vi "Teleop.vi"(10 "Match Info":T2={"Autonomous Elapsed Seconds"=0.0, "TeleOp Elapsed Seconds"=0.0, "Disabled Elapsed Seconds"=0.0, "Visited Autonomous"=FALSE, "Visited TeleOp"=FALSE, "Visited Disabled"=FALSE, "Autonomous Settings"={"Autonomous Style"=enum."Independent", "VI Refnum"=refnum}}, 11 "Call Context":T1) -> ()   [LabVIEW 2013]
doc: "This VI is called for each TeleOp packet received from the DS where the robot is not disabled. It is often used to read from the joysticks and update I/O or to update setpoints for timed control loops. It should complete and return within 20 milliseconds or it may miss DS packets."
uses:
  <vilib>/Rock Robotics/WPI/DriverStation/WPI_DriverStationMatch Info.ctl
  <vilib>/Rock Robotics/WPI/DriverStation/WPI_DriverStationDerivedRobotMode.ctl
  Robot Global Data.vi
  <vilib>/Rock Robotics/WPI/Solenoid/Deprecated/WPI_SolenoidSetBool.vi
  <vilib>/Rock Robotics/WPI/Joystick/WPI_JoystickGetSetRefNum.vi
  <vilib>/Rock Robotics/WPI/Compressor/WPI_CompressorGetSetRefNum.vi
  <vilib>/Rock Robotics/WPI/RobotDrive/WPI_RobotDriveGetSetRefNum.vi
panel:
  in  "Uncock tension":dbl=0.15
  in  "Manual Tension Power":dbl=0.7
  out "hot?":bool
  out "shouldTurnRight":bool
  in  "Ball In Delay":dbl=1.75
  out "Arm Half Out":bool
  out "Timings":cluster{"Call Name":string, "Delta (ms)":u32}[](array[cluster])
  out "Right":dbl
  out "Left":dbl
  out "Encoders":dbl
  out "Angular Rate":dbl
  out "Angle":dbl
  out "Numeric 1":dbl(slide) scale=0.0..100.0
  out "Boolean 2":bool
  out "Boolean 1":bool
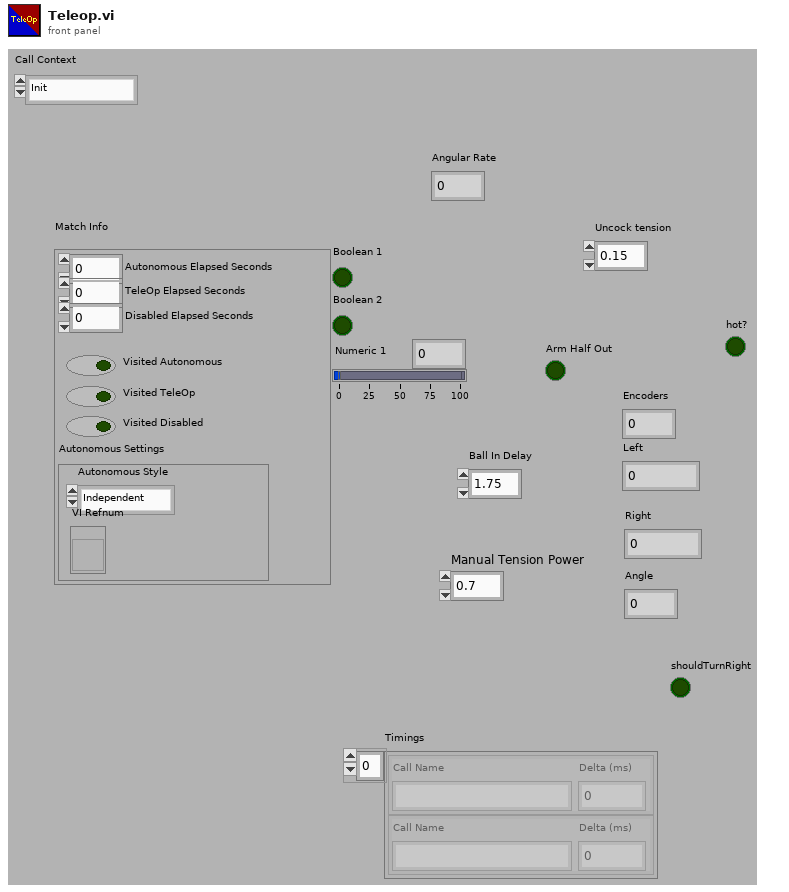
[diagram p1: front panel]
types:
  T1 = typedef "WPI_DriverStationDerivedRobotMode.ctl" = enum16{"Init", "Execute", "Stop"}
  T2 = typedef "WPI_DriverStationMatch Info.ctl" = cluster{"Autonomous Elapsed Seconds":dbl, "TeleOp Elapsed Seconds":dbl, "Disabled Elapsed Seconds":dbl, "Visited Autonomous":bool, "Visited TeleOp":bool, "Visited Disabled":bool, "Autonomous Settings":cluster{"Autonomous Style":enum16{"Iterative", "Independent"}, "VI Refnum":refnum<vi>}}
  T3 = typedef "WPI_JoystickDevRef.ctl" = cluster{"Device":T4}
  T4 = typedef "WPI_JoystickDeviceEnum.ctl" = enum16{"USB 1", "USB 2", "USB 3", "USB 4", "Kinect 1", "Kinect 2"}
  T5 = typedef "WPI_RobotDriveDevRef.ctl" = cluster{"DevStatus":errorcluster, "Motors[]":T6[], "Square Inputs":bool, "Max Output":dbl, "Isochronous":bool}
  T6 = typedef "WPI_MotorControlDeviceRef.ctl" = cluster{"DeviceStatus":errorcluster, "Type":enum16{"PWM", "CAN"}, "PWM":cluster{"Digital Module":T7, "PWM Channel":T8, "DeadBand":T9}, "CAN":cluster{"Device Number":u8, "Control Mode":T10, "Semaphore":T11, "Max Vout":dbl}, "Invert":bool, "TransformRef":T12, "InvTransformRef":T12}
  T7 = typedef "FPGA_TypedefDigitalModule.ctl" = enum16{"Digital Module 1", "Digital Module 2"}
  T8 = typedef "FPGA_DIOPWMChannel.ctl" = enum8{"PWM 1", "PWM 2", "PWM 3", "PWM 4", "PWM 5", "PWM 6", "PWM 7", "PWM 8", "PWM 9", "PWM 10", "Invalid"}
  T9 = typedef "WPI_PWMDeadband.ctl" = cluster{"Name":string, "maxPositivePwm":i32, "minPositivePwm":i32, "centerPwm":i32, "maxNegativePwm":i32, "minNegativePwm":i32, "angularRange":u16}
  T10 = typedef "WPI_CANJaguar_ControlMode.ctl" = enum8{"Percent VBus", "Current", "Speed", "Position", "Voltage"}
  T11 = typedef "Semaphore RefNum" = refnum<k1>
  T12 = typedef "WPI_PWMTransform_ConPane.ctl" = refnum<vi>
  T13 = typedef "WPI_JoystickButtonState.ctl" = cluster{"Button 1":bool, "Button 2":bool, "Button 3":bool, "Button 4":bool, "Button 5":bool, "Button 6":bool, "Button 7":bool, "Button 8":bool, "Button 9":bool, "Button 10":bool, "Button 11":bool, "Button 12":bool}
  T14 = cluster{"axis 1 (x)":dbl, "axis 2 (y)":dbl, "axis 3 (throttle)":dbl, "axis 4":dbl, "axis 5":dbl, "axis 6":dbl}
  T15 = typedef "WPI_CompressorDevRef.ctl" = cluster{"DevStatus":errorcluster, "DigitalInputDevRef":T16, "RelayDevRef":T18}
  T16 = typedef "WPI_DigitalInputDevRef.ctl" = cluster{"DevStatus":errorcluster, "DIO Channel":T17, "Digital Module":T7}
  T17 = typedef "FPGA_DIOChannel.ctl" = enum8{"DIO 1", "DIO 2", "DIO 3", "DIO 4", "DIO 5", "DIO 6", "DIO 7", "DIO 8", "DIO 9", "DIO 10", "DIO 11", "DIO 12", "DIO 13", "DIO 14", "Invalid"}
  T18 = typedef "WPI_RelayDevRef.ctl" = cluster{"DevStatus":errorcluster, "Relay Channel":T19, "Digital Module":T7, "Relay Direction":T20}
  T19 = typedef "FPGA_DIORelayChannel.ctl" = enum8{"Relay 1", "Relay 2", "Relay 3", "Relay 4", "Relay 5", "Relay 6", "Relay 7", "Relay 8", "Invalid"}
  T20 = typedef "WPI_RelayDirection.ctl" = enum16{"Both directions", "Forward only", "Reverse only"}
  T21 = typedef "WPI_SolenoidDevRef.ctl" = cluster{"DevStatus":errorcluster, "Solenoid Module":T22, "Forward Solenoid Channel":T23, "Reverse Solenoid Channel":T23}
  T22 = typedef "FPGA_TypedefSolenoidModule.ctl" = enum16{"Solenoid Module 1", "Solenoid Module 2"}
  T23 = typedef "WPI_SolenoidChannel.ctl" = enum8{"Solenoid 1", "Solenoid 2", "Solenoid 3", "Solenoid 4", "Solenoid 5", "Solenoid 6", "Solenoid 7", "Solenoid 8", "Invalid"}
  T24 = typedef "WPI_GyroDevRef.ctl" = cluster{"DevStatus":errorcluster, "Analog Module":T25, "Analog Channel":T26, "Offset":dbl, "Gain (VoltsPerDegree/Second)":dbl}
  T25 = typedef "FPGA_TypedefAnalogModule.ctl" = enum16{"Analog Module 1", "Analog Module 2"}
  T26 = typedef "FPGA_AIChannel.ctl" = enum8{"AI 1", "AI 2", "AI 3", "AI 4", "AI 5", "AI 6", "AI 7", "AI 8", "Invalid"}
  T27 = typedef "WPI_AnalogChannelDevRef.ctl" = cluster{"DevStatus":errorcluster, "Analog Module":T25, "Analog Channel":T26}
  T28 = typedef "WPI_EncoderDevRef.ctl" = cluster{"DevStatus":errorcluster, "EncoderIndex":T29, "CounterIndex":T30, "DistancePerCount":dbl, "Decoding Type":T31}
  T29 = typedef "FPGA_EncoderIdx.ctl" = enum8{"Enc 0", "Enc 1", "Enc 2", "Enc 3", "Invalid"}
  T30 = typedef "FPGA_CounterCtrSystemIndex.ctl" = enum8{"Ctr 0", "Ctr 1", "Ctr 2", "Ctr 3", "Ctr 4", "Ctr 5", "Ctr 6", "Ctr 7", "Invalid"}
  T31 = typedef "WPI_EncoderType.ctl" = enum16{"1x", "2x", "4x"}
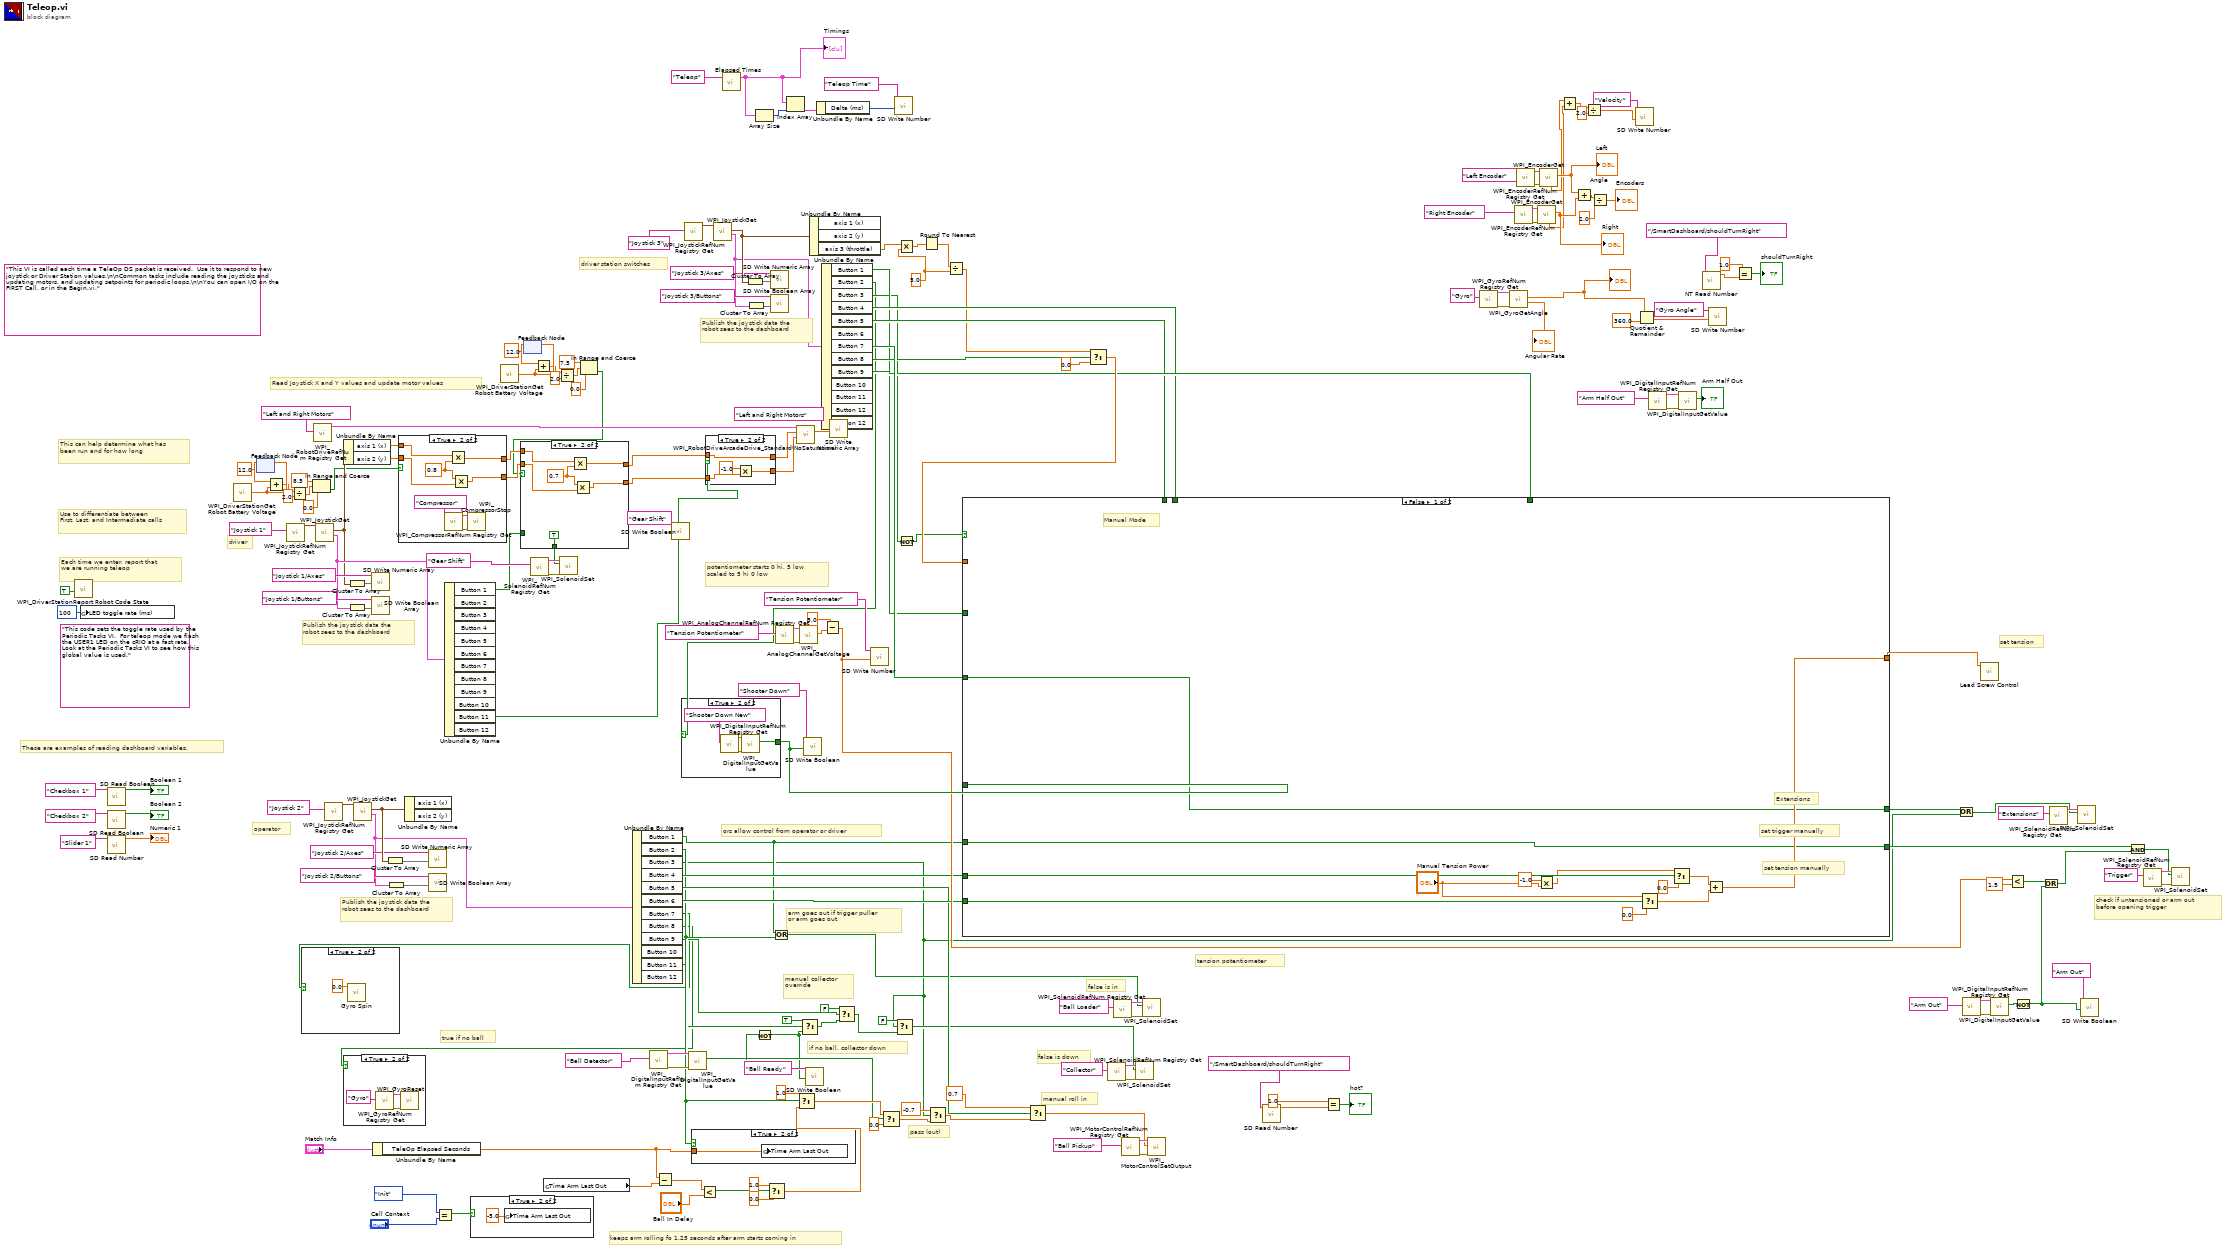
[diagram p0: block diagram]
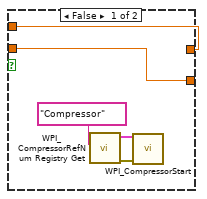
[diagram p4: hidden frame]
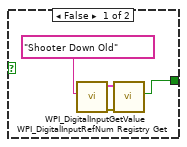
[diagram p7: hidden frame]
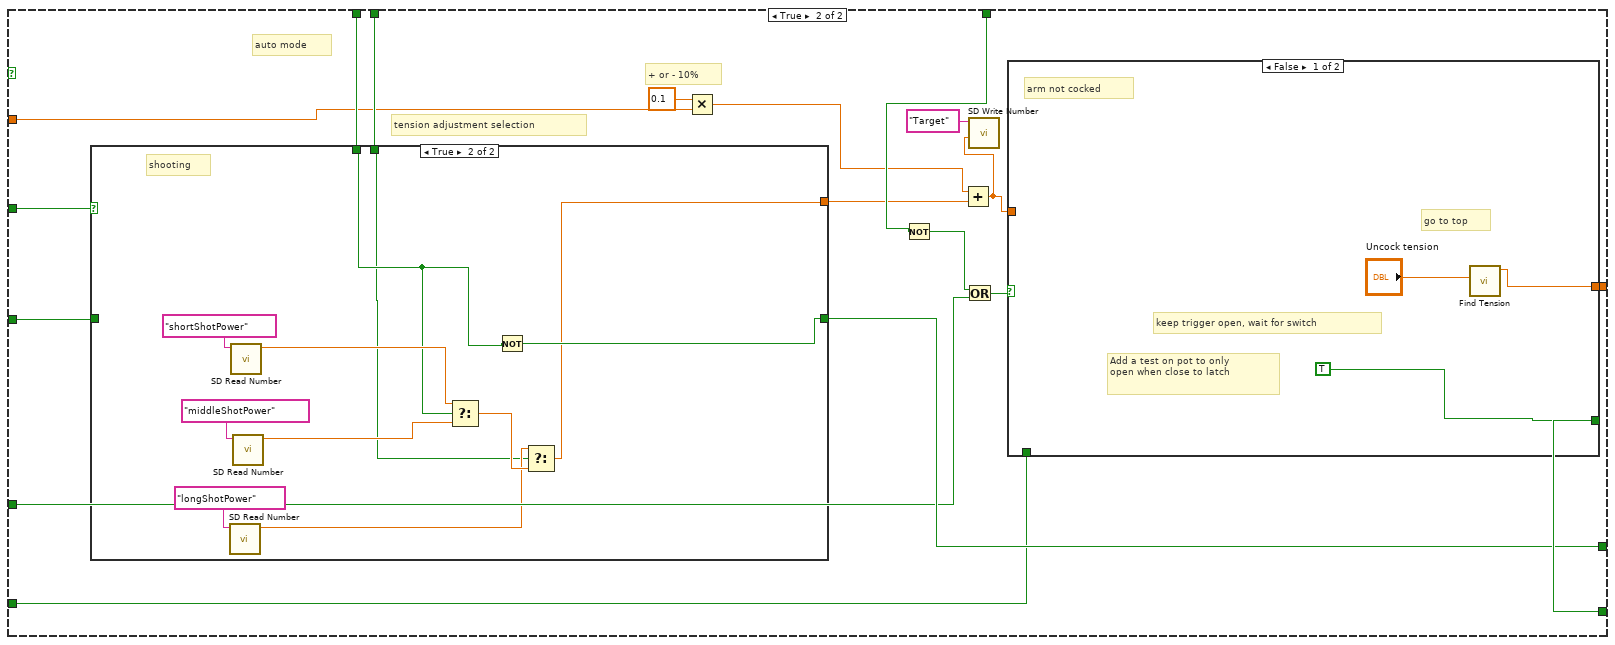
[diagram p10: hidden frame]
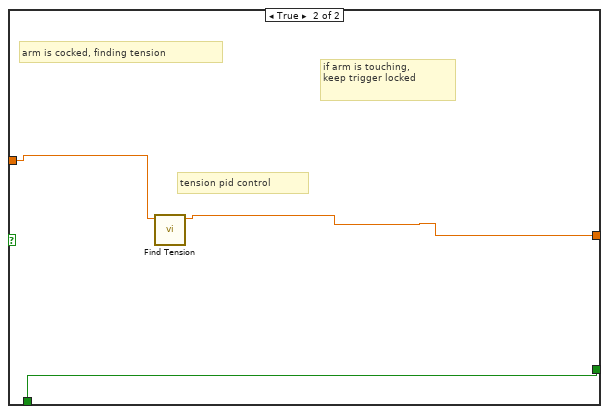
[diagram p11: hidden frame]
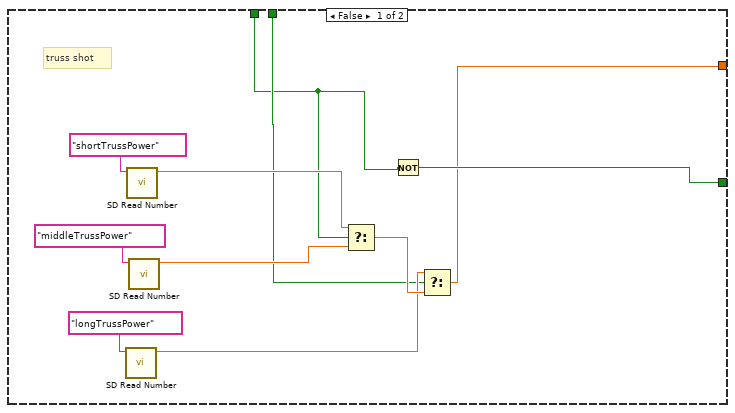
[diagram p12: hidden frame]
diagram:
  w26 = 5.0
  (unwired) "This code sets the toggle rate used by the Periodic Tasks VI.  For teleop mode we flash the USER1 LED on the cRIO at a fast rate.  Look at the Periodic Tasks VI to see how this global value is used."
  (unwired) "This VI is called each time a TeleOp DS packet is received.  Use it to respond to new joystick or Driver Station values.\n\nCommon tasks include reading the joysticks and updating motors, and updating setpoints for periodic loops.\n\nYou can open I/O on the FIRST Call, or in the Begin.vi."
  # "tension potentiometer"
  # "if no ball, collector down"
  # "manual collector \noverride"
  # "manual roll in"
  # "pass (out)"
  # "arm goes out if trigger puller\nor arm goes out"
  # "false is in"
  # "false is down"
  # "true if no ball"
  # "set tension"
  # "driver station switches"
  # "operator"
  # "driver"
  # "ors allow control from operator or driver"
  # "keeps arm rolling fo 1.25 seconds after arm starts coming in"
  # "potentiometer starts 0 hi, 5 low\nscaled to 5 hi 0 low"
  # "check if untensioned or arm out \nbefore opening trigger"
  # "Publish the joystick data the\nrobot sees to the dashboard"
  # "Publish the joystick data the\nrobot sees to the dashboard"
  # "These are examples of reading dashboard variables."
  # "Publish the joystick data the\nrobot sees to the dashboard"
  # "Each time we enter, report that\nwe are running teleop"
  # "Use to differentiate between\nFirst, Last, and Intermediate calls"
  # "This can help determine what has\nbeen run and for how long"
  # "Read Joystick X and Y values and update motor values"
  n1 = call <vilib>:"WPI_DriverStationReport Robot Code State.vi"("TeleOp"=TRUE ("Autonomous")) -> ()  [unwired: 10 in, 1 out]
  n2 = global write "Robot Global Data.vi" "LED toggle rate (ms)"(u32 100 ("LED ms toggle rate")) -> ()
  n3 = call <vilib>:"SD Read Boolean.vi"("Name"="Checkbox 1" ("refnum name")) -> ("Boolean"=→"Boolean 1":bool)  [unwired: 8 in, 2 out]
  n4 = call <vilib>:"SD Read Boolean.vi"("Name"="Checkbox 2" ("refnum name")) -> ("Boolean"=→"Boolean 2":bool)  [unwired: 8 in, 2 out]
  n5 = call <vilib>:"SD Read Number.vi"("Name"="Slider 1" ("refnum name")) -> ("Numeric"=→"Numeric 1":dbl)  [unwired: 8 in, 2 out]
  n6 = call <vilib>:"WPI_DriverStationGet Robot Battery Voltage.vi"() -> ("robot battery voltage"=w24:dbl)  [unwired: 14 in, 1 out]
  n7 = feedback-in #1(w24) -> ()
  n8 = feedback #1(12.0 ("robot battery voltage")) -> (w25:dbl)
  n9 = Add(x=w25, y=w24) -> (x+y=w23:dbl)
  n10 = call <vilib>:"WPI_JoystickRefNum Registry Get.vi"("refnum name"="Joystick 1") -> ("JoystickDevRef"=w204:T3)  [unwired: 1 in, 9 out]
  n11 = Divide(x=w23, y=2.0) -> (x/y=w12:dbl)
  n12 = In Range and Coerce(upper limit=8.5, x=w12, lower limit=0.0) -> (In Range?=w51:bool)  [unwired: 1 out]
  n13 = call <vilib>:"WPI_RobotDriveRefNum Registry Get.vi"("refnum name"="Left and Right Motors") -> ("RobotDriveDevRef"=w206:T5)  [unwired: 1 in, 9 out]
  n14 = call <vilib>:"WPI_JoystickGet.vi"("JoystickDevRef"=w204) -> ("Buttons"=w189:T13, "Axes"=w54:T14)  [unwired: 1 in, 4 out]
  n15 = call <vilib>:"WPI_JoystickRefNum Registry Get.vi"("refnum name"="Joystick 2") -> ("JoystickDevRef"=w187:T3)  [unwired: 1 in, 9 out]
  n16 = Unbundle By Name(w54) -> ("axis 1 (x)"=w52:dbl, "axis 2 (y)"=w53:dbl)
  n17 = Cluster To Array(cluster=w54) -> (array=w199:dbl[])
  n18 = Cluster To Array(cluster=w189) -> (array=w201:bool[])
  n19 = call <vilib>:"WPI_JoystickGet.vi"("JoystickDevRef"=w187) -> ("Buttons"=w181:T13, "Axes"=w184:T14)  [unwired: 1 in, 4 out]
  n20 = call <vilib>:"SD Write Numeric Array.vi"("Numeric Array"=w199, "Name"="Joystick 1/Axes") -> ()  [unwired: 8 in, 2 out]
  n21 = call <vilib>:"SD Write Boolean Array.vi"("Boolean Array"=w201, "Name"="Joystick 1/Buttons") -> ()  [unwired: 8 in, 2 out]
  n22 = Unbundle By Name("Match Info") -> ("TeleOp Elapsed Seconds"=w134:dbl)
  n23 = Cluster To Array(cluster=w184) -> (array=w183:dbl[])
  n24 = Cluster To Array(cluster=w181) -> (array=w186:bool[])
  n25 = case shown="True" w51 {
    tunnel: [w213 w217] -> w50
    tunnel: w53 -> [w213 w220]
    tunnel: [w212 w218] -> w49
    tunnel: w52 -> [w212 w221]
    frame False {
      n26 = call <vilib>:"WPI_CompressorRefNum Registry Get.vi"("refnum name"="Compressor") -> ("error out"=w210:errorcluster, "CompressorDevRef"=w209:T15)  [unwired: 9 in]
      n27 = call <vilib>:"WPI_CompressorStart.vi"("error in (no error)"=w210, "CompressorDevRef"=w209) -> ()  [unwired: 8 in, 2 out]
    }
    frame True {
      w219 = 0.8
      n28 = call <vilib>:"WPI_CompressorRefNum Registry Get.vi"("refnum name"="Compressor") -> ("error out"=w215:errorcluster, "CompressorDevRef"=w216:T15)  [unwired: 9 in]
      n29 = Multiply(x=w221, y=w219) -> (x*y=w218:dbl)
      n30 = Multiply(x=w219, y=w220) -> (x*y=w217:dbl)
      n31 = call <vilib>:"WPI_CompressorStop.vi"("error in (no error)"=w215, "CompressorDevRef"=w216) -> ()  [unwired: 8 in, 2 out]
    }
  }
  n32 = Unbundle By Name(w184) -> ()  [unwired: 2 out]
  n33 = call <vilib>:"SD Write Numeric Array.vi"("Numeric Array"=w183, "Name"="Joystick 2/Axes") -> ()  [unwired: 8 in, 2 out]
  n34 = call <vilib>:"SD Write Boolean Array.vi"("Boolean Array"=w186, "Name"="Joystick 2/Buttons") -> ()  [unwired: 8 in, 2 out]
  n35 = Equal?(x=WPI_DriverStationDerivedRobotMode."Init" ("Call Context"), y="Call Context") -> (x = y?=w8:bool)
  n36 = Unbundle By Name(w189) -> ("Button 1"=w30:bool, "Button 11"=w110:bool)  [unwired: 10 out]
  n37 = case shown="True" w8 {
    frame False {
    }
    frame True {
      n38 = global write "Robot Global Data.vi" "Time Arm Last Out"(-5.0 ("Time Arm Last Out")) -> ()
    }
  }
  n39 = call <vilib>:"WPI_DriverStationGet Robot Battery Voltage.vi"() -> ("robot battery voltage"=w17:dbl)  [unwired: 14 in, 1 out]
  n40 = feedback #2(12.0 ("robot battery voltage")) -> (w18:dbl)
  n41 = feedback-in #2(w17) -> ()
  n42 = call <vilib>:"WPI_SolenoidRefNum Registry Get.vi"("refnum name"="Gear Shift") -> ("error out"=w172:errorcluster, "SolenoidDevRef"=w171:T21)  [unwired: 9 in]
  n43 = Add(x=w18, y=w17) -> (x+y=w16:dbl)
  n44 = global read "Robot Global Data.vi" "Time Arm Last Out"() -> (w136:dbl)
  n45 = Divide(x=w16, y=2.0) -> (x/y=w11:dbl)
  n46 = In Range and Coerce(upper limit=7.5, x=w11, lower limit=0.0) -> (In Range?=w13:bool)  [unwired: 1 out]
  n47 = case shown="True" w13 {
    tunnel: [w225 w227] -> w47
    tunnel: w50 -> [w225 w230]
    tunnel: [w224 w228] -> w48
    tunnel: w49 -> [w224 w231]
    tunnel: [w223 TRUE] -> w31
    tunnel: w30 -> [w223 _]
    frame False {
    }
    frame True {
      w229 = 0.7
      n48 = Multiply(x=w231, y=w229) -> (x*y=w228:dbl)
      n49 = Multiply(x=w229, y=w230) -> (x*y=w227:dbl)
    }
  }
  n50 = call-poly <vilib>:"WPI_SolenoidSet.vi"("error in (no error)"=w172, "Value"=w31, "SolenoidDevRef"=w171) -> ()  [unwired: 7 in, 2 out]
  n51 = Unbundle By Name(w181) -> ("Button 1"=w93:bool, "Button 2"=w92:bool, "Button 3"=w32:bool, "Button 4"=w102:bool, "Button 5"=w97:bool, "Button 6"=w106:bool, "Button 7"=w84:bool, "Button 8"=w57:bool, "Button 9"=w89:bool, "Button 11"=w90:bool)  [unwired: 2 out]
  n52 = case shown="True" w84 {
    frame False {
    }
    frame True {
      n53 = call "Gyro Spin.vi"("Desired Angle"=0.0) -> ()  [unwired: 10 in, 1 out]
    }
  }
  n54 = case shown="True" w57 {
    frame False {
    }
    frame True {
      n55 = call <vilib>:"WPI_GyroRefNum Registry Get.vi"("refnum name"="Gyro") -> ("error out"=w234:errorcluster, "GyroDevRef"=w233:T24)  [unwired: 9 in]
      n56 = call <vilib>:"WPI_GyroReset.vi"("error in (no error)"=w234, "GyroDevRef"=w233) -> ()  [unwired: 8 in, 2 out]
    }
  }
  n57 = call <vilib>:"WPI_DigitalInputRefNum Registry Get.vi"("refnum name"="Ball Detector") -> ("error out"=w103:errorcluster, "DigitalInputDevRef"=w104:T16)  [unwired: 9 in]
  n58 = Subtract(x=w134, y=w136) -> (x-y=w135:dbl)
  n59 = call <vilib>:"SD Write Boolean.vi"("Name"="Gear Shift") -> ()  [unwired: 9 in, 2 out]
  n60 = call <vilib>:"WPI_JoystickRefNum Registry Get.vi"("refnum name"="Joystick 3") -> ("JoystickDevRef"=w179:T3)  [unwired: 1 in, 9 out]
  n61 = call <vilib>:"WPI_DigitalInputGetValue.vi"("error in (no error)"=w103, "DigitalInputDevRef"=w104) -> ("Value"=w4:bool)  [unwired: 7 in, 2 out]
  n62 = case shown="True" w92 {
    tunnel: w134 -> [_ w236]
    frame False {
    }
    frame True {
      n63 = global write "Robot Global Data.vi" "Time Arm Last Out"(w236) -> ()
    }
  }
  n64 = Less?(x=w135, y="Ball In Delay") -> (x < y?=w146:bool)
  n65 = case shown="True" w110 {
    tunnel: w48 -> [w238 w239]
    tunnel: [w237 w241] -> w109
    tunnel: [w238 w239] -> w108
    tunnel: w47 -> [w237 w240]
    frame False {
    }
    frame True {
      n66 = Multiply(x=-1.0 ("y"), y=w240) -> (x*y=w241:dbl)
    }
  }
  n67 = call <vilib>:"WPI_JoystickGet.vi"("JoystickDevRef"=w179) -> ("Buttons"=w173:T13, "Axes"=w176:T14)  [unwired: 1 in, 4 out]
  n68 = call "Elapsed Times.vi"("Call Name"="Teleop") -> ("Timings"=w121:cluster{"Call Name":string, "Delta (ms)":u32}[])  [unwired: 2 in]
  "Timings" <- w121
  n69 = Cluster To Array(cluster=w176) -> (array=w175:dbl[])
  n70 = Cluster To Array(cluster=w173) -> (array=w178:bool[])
  n71 = Array Size(array=w121) -> (size(s)=w120:i32)
  n72 = Not(x=w4) -> (.not. x?=w1:bool)
  n73 = Select(t=1.0, s=w146, f=0.0) -> (s? t:f=w6:dbl)
  n74 = call <vilib>:"SD Write Numeric Array.vi"("Numeric Array"=w175, "Name"="Joystick 3/Axes") -> ()  [unwired: 8 in, 2 out]
  n75 = call <vilib>:"SD Write Boolean Array.vi"("Boolean Array"=w178, "Name"="Joystick 3/Buttons") -> ()  [unwired: 8 in, 2 out]
  n76 = Or(x=w93, y=w92) -> (x .or. y?=w91:bool)
  n77 = call <vilib>:"WPI_AnalogChannelRefNum Registry Get.vi"("refnum name"="Tension Potentiometer") -> ("error out"=w169:errorcluster, "AIDeviceRef"=w168:T27)  [unwired: 9 in]
  n78 = Index Array(array=w121, index=w120) -> (element=w124:cluster{"Call Name":string, "Delta (ms)":u32})
  n79 = call <vilib>:"WPI_RobotDriveArcadeDrive_Standard(NoSaturation).vi"("Y axis value"=w109, "X axis value"=w108, "RobotDriveDevRef"=w206) -> ("Motor Values"=w196:dbl[])  [unwired: 1 in, 7 out]
  n80 = Select(t=1.0, s=w92, f=w6) -> (s? t:f=w5:dbl)
  n81 = call <vilib>:"WPI_AnalogChannelGetVoltage.vi"("error in (no error)"=w169, "AIDeviceRef"=w168) -> ("Voltage"=w138:dbl)  [unwired: 7 in, 2 out]
  n82 = Select(t=TRUE, s=w90, f=w1) -> (s? t:f=w86:bool)
  n83 = call <vilib>:"SD Write Boolean.vi"("Boolean"=w1, "Name"="Ball Ready") -> ()  [unwired: 8 in, 2 out]
  n84 = Unbundle By Name(w176) -> ("axis 3 (throttle)"=w28:dbl)  [unwired: 2 out]
  n85 = Unbundle By Name(w124) -> ("Delta (ms)"=w123:u32)
  n86 = Unbundle By Name(w173) -> ("Button 1"=w117:bool, "Button 2"=w107:bool, "Button 3"=w115:bool, "Button 4"=w119:bool, "Button 5"=w118:bool, "Button 7"=w148:bool, "Button 8"=w133:bool, "Button 9"=w126:bool)  [unwired: 5 out]
  n87 = case shown="True" w107 {
    tunnel: [w243 w247] -> w151
    frame False {
      n88 = call <vilib>:"WPI_DigitalInputRefNum Registry Get.vi"("refnum name"="Shooter Down Old") -> ("error out"=w246:errorcluster, "DigitalInputDevRef"=w245:T16)  [unwired: 9 in]
      n89 = call <vilib>:"WPI_DigitalInputGetValue.vi"("error in (no error)"=w246, "DigitalInputDevRef"=w245) -> ("Value"=w243:bool)  [unwired: 7 in, 2 out]
    }
    frame True {
      n90 = call <vilib>:"WPI_DigitalInputRefNum Registry Get.vi"("refnum name"="Shooter Down New") -> ("error out"=w250:errorcluster, "DigitalInputDevRef"=w249:T16)  [unwired: 9 in]
      n91 = call <vilib>:"WPI_DigitalInputGetValue.vi"("error in (no error)"=w250, "DigitalInputDevRef"=w249) -> ("Value"=w247:bool)  [unwired: 7 in, 2 out]
    }
  }
  n92 = call <vilib>:"SD Write Boolean.vi"("Boolean"=w151, "Name"="Shooter Down") -> ()  [unwired: 8 in, 2 out]
  n93 = Subtract(x=5.0, y=w138) -> (x-y=w130:dbl)
  n94 = call <vilib>:"SD Write Numeric Array.vi"("Numeric Array"=w196, "Name"="Left and Right Motors") -> ()  [unwired: 8 in, 2 out]
  n95 = Select(t=FALSE, s=w89, f=w86) -> (s? t:f=w46:bool)
  n96 = call <vilib>:"SD Write Number.vi"("Numeric"=w130, "Name"="Tension Potentiometer") -> ()  [unwired: 8 in, 2 out]
  n97 = Select(t=w5, s=w4, f=0.0) -> (s? t:f=w99:dbl)
  n98 = call <vilib>:"SD Write Number.vi"("Numeric"=w123, "Name"="Teleop Time") -> ()  [unwired: 8 in, 2 out]
  n99 = Select(t=FALSE, s=w32, f=w46) -> (s? t:f=w45:bool)
  n100 = Multiply(x=w28, y=w26) -> (x*y=w27:dbl)
  n101 = Not(x=w115) -> (.not. x?=w116:bool)
  n102 = Round To Nearest(number=w27) -> (nearest integer value=w29:dbl)
  n103 = Select(t=-0.7, s=w32, f=w99) -> (s? t:f=w96:dbl)
  n104 = Divide(x=w29, y=w26) -> (x/y=w7:dbl)
  n105 = Select(t=0.7, s=w97, f=w96) -> (s? t:f=w94:dbl)
  n106 = Select(t=w7, s=w133, f=0.0) -> (s? t:f=w131:dbl)
  n107 = case shown="False" w116 {
    tunnel: w102 -> [w261 _]
    tunnel: w106 -> [w262 _]
    tunnel: w93 -> [w255 w276]
    tunnel: w151 -> [_ w266]
    tunnel: w131 -> [_ w273]
    tunnel: w148 -> [w254 w277]
    tunnel: [w255 w280] -> w143
    tunnel: [w256 w279] -> w105
    tunnel: [w254 w278] -> w34
    tunnel: w118 -> [_ w274]
    tunnel: w119 -> [_ w275]
    tunnel: w126 -> [_ w268]
    tunnel: w117 -> [_ w269]
    frame False {
      # "Extensions"
      # "set tension manually"
      # "set trigger manually"
      # "Manual Mode"
      n108 = Multiply(x=-1.0, y="Manual Tension Power") -> (x*y=w251:dbl)
      n109 = Select(t="Manual Tension Power", s=w262, f=0.0) -> (s? t:f=w257:dbl)
      n110 = Select(t=w251, s=w261, f=0.0) -> (s? t:f=w258:dbl)
      n111 = Add(x=w258, y=w257) -> (x+y=w256:dbl)
    }
    frame True {
      # "+ or - 10%"
      # "tension adjustment selection"
      # "auto mode"
      n112 = case shown="True" w269 {
        tunnel: w277 -> [_ _]
        tunnel: [w297 w301] -> w278
        tunnel: w275 -> [w288 w298]
        tunnel: w274 -> [w287 w299]
        tunnel: [w289 w300] -> w264
        frame False {
          # "truss shot"
          n113 = call <vilib>:"SD Read Number.vi"("Name"="longTrussPower") -> ("Numeric"=w290:dbl)  [unwired: 8 in, 2 out]
          n114 = call <vilib>:"SD Read Number.vi"("Name"="shortTrussPower") -> ("Numeric"=w292:dbl)  [unwired: 8 in, 2 out]
          n115 = call <vilib>:"SD Read Number.vi"("Name"="middleTrussPower") -> ("Numeric"=w293:dbl)  [unwired: 8 in, 2 out]
          n116 = Select(t=w292, s=w287, f=w293) -> (s? t:f=w291:dbl)
          n117 = Not(x=w287) -> (.not. x?=w297:bool)
          n118 = Select(t=w290, s=w288, f=w291) -> (s? t:f=w289:dbl)
        }
        frame True {
          # "shooting"
          n119 = call <vilib>:"SD Read Number.vi"("Name"="longShotPower") -> ("Numeric"=w302:dbl)  [unwired: 8 in, 2 out]
          n120 = call <vilib>:"SD Read Number.vi"("Name"="shortShotPower") -> ("Numeric"=w304:dbl)  [unwired: 8 in, 2 out]
          n121 = call <vilib>:"SD Read Number.vi"("Name"="middleShotPower") -> ("Numeric"=w305:dbl)  [unwired: 8 in, 2 out]
          n122 = Select(t=w304, s=w299, f=w305) -> (s? t:f=w303:dbl)
          n123 = Not(x=w299) -> (.not. x?=w301:bool)
          n124 = Select(t=w302, s=w298, f=w303) -> (s? t:f=w300:dbl)
        }
      }
      n125 = Multiply(x=0.1, y=w273) -> (x*y=w263:dbl)
      n126 = Not(x=w268) -> (.not. x?=w265:bool)
      n127 = Add(x=w263, y=w264) -> (x+y=w270:dbl)
      n128 = Or(x=w265, y=w266) -> (x .or. y?=w267:bool)
      n129 = call <vilib>:"SD Write Number.vi"("Numeric"=w270, "Name"="Target") -> ()  [unwired: 8 in, 2 out]
      n130 = case shown="False" w267 {
        tunnel: [w282 w284] -> w279
        tunnel: [TRUE w286] -> w280
        tunnel: w270 -> [_ w285]
        tunnel: w276 -> [_ w286]
        frame False {
          # "go to top"
          # "Add a test on pot to only\nopen when close to latch"
          # "keep trigger open, wait for switch"
          # "arm not cocked"
          n131 = call "Find Tension.vi"("Desired Tension"="Uncock tension") -> ("Motor Output"=w282:dbl)  [unwired: 9 in, 1 out]
        }
        frame True {
          # "tension pid control"
          # "arm is cocked, finding tension"
          # "if arm is touching,\nkeep trigger locked"
          n132 = call "Find Tension.vi"("Desired Tension"=w285) -> ("Motor Output"=w284:dbl)  [unwired: 9 in, 1 out]
        }
      }
    }
  }
  n133 = call <vilib>:"WPI_SolenoidRefNum Registry Get.vi"("refnum name"="Collector") -> ("error out"=w127:errorcluster, "SolenoidDevRef"=w129:T21)  [unwired: 9 in]
  n134 = call <vilib>:"WPI_SolenoidRefNum Registry Get.vi"("refnum name"="Ball Loader") -> ("error out"=w156:errorcluster, "SolenoidDevRef"=w159:T21)  [unwired: 9 in]
  n135 = call <vilib>:"WPI_MotorControlRefNum Registry Get.vi"("refnum name"="Ball Pickup") -> ("error out"=w155:errorcluster, "MotorControlDevRef"=w163:T6)  [unwired: 9 in]
  n136 = call-poly <vilib>:"WPI_SolenoidSet.vi"("error in (no error)"=w127, "Value"=w45, "SolenoidDevRef"=w129) -> ()  [unwired: 7 in, 2 out]
  n137 = call-poly <vilib>:"WPI_SolenoidSet.vi"("error in (no error)"=w156, "Value"=w91, "SolenoidDevRef"=w159) -> ()  [unwired: 7 in, 2 out]
  n138 = call <vilib>:"WPI_MotorControlSetOutput.vi"("error in (no error)"=w155, "Output"=w94, "MotorControlDevRef"=w163) -> ()  [unwired: 6 in, 3 out]
  n139 = call <vilib>:"SD Read Number.vi"("Name"="/SmartDashboard/shouldTurnRight") -> ("Numeric"=w42:dbl)  [unwired: 8 in, 2 out]
  n140 = Equal?(x=1.0, y=w42) -> (x = y?=→"hot?":bool)
  n141 = call <vilib>:"WPI_GyroRefNum Registry Get.vi"("refnum name"="Gyro") -> ("error out"=w83:errorcluster, "GyroDevRef"=w82:T24)  [unwired: 9 in]
  n142 = call <vilib>:"WPI_GyroGetAngle.vi"("error in (no error)"=w83, "GyroDevRef"=w82) -> ("Angular Rate"=→"Angular Rate":dbl, "Angle"=w39:dbl)  [unwired: 6 in, 2 out]
  "Angle" <- w39
  n143 = call <vilib>:"WPI_EncoderRefNum Registry Get.vi"("refnum name"="Right Encoder") -> ("error out"=w76:errorcluster, "EncoderDevRef"=w75:T28)  [unwired: 9 in]
  n144 = call <vilib>:"WPI_EncoderRefNum Registry Get.vi"("refnum name"="Left Encoder") -> ("error out"=w79:errorcluster, "EncoderDevRef"=w78:T28)  [unwired: 9 in]
  n145 = call <vilib>:"WPI_EncoderGet.vi"("error in (no error)"=w76, "EncoderDevRef"=w75) -> ("Distance"=w72:dbl, "Rate"=w62:dbl)  [unwired: 4 in, 4 out]
  "Right" <- w72
  n146 = call <vilib>:"WPI_EncoderGet.vi"("error in (no error)"=w79, "EncoderDevRef"=w78) -> ("Distance"=w70:dbl, "Rate"=w61:dbl)  [unwired: 4 in, 4 out]
  "Left" <- w70
  n147 = Add(x=w61, y=w62) -> (x+y=w64:dbl)
  n148 = Add(x=w70, y=w72) -> (x+y=w73:dbl)
  n149 = Divide(x=w64, y=2.0) -> (x/y=w60:dbl)
  n150 = Divide(x=w73, y=2.0) -> (x/y=→"Encoders":dbl)
  n151 = call <vilib>:"SD Write Number.vi"("Numeric"=w60, "Name"="Velocity") -> ()  [unwired: 8 in, 2 out]
  n152 = Quotient & Remainder(x=w39, y=360.0) -> (floor(x/y)=w37:dbl)  [unwired: 1 out]
  n153 = call <vilib>:"WPI_DigitalInputRefNum Registry Get.vi"("refnum name"="Arm Half Out") -> ("error out"=w112:errorcluster, "DigitalInputDevRef"=w114:T16)  [unwired: 9 in]
  n154 = call <vilib>:"WPI_DigitalInputGetValue.vi"("error in (no error)"=w112, "DigitalInputDevRef"=w114) -> ("Value"=→"Arm Half Out":bool)  [unwired: 7 in, 2 out]
  n155 = call <vilib>:"NT Read Number.vi"("Name"="/SmartDashboard/shouldTurnRight") -> ("Numeric"=w68:dbl)  [unwired: 9 in, 1 out]
  n156 = call <vilib>:"SD Write Number.vi"("Numeric"=w37, "Name"="Gyro Angle") -> ()  [unwired: 8 in, 2 out]
  n157 = Equal?(x=1.0, y=w68) -> (x = y?=→"shouldTurnRight":bool)
  n158 = Or(x=w34, y=w32) -> (x .or. y?=w33:bool)
  n159 = call <vilib>:"WPI_DigitalInputRefNum Registry Get.vi"("refnum name"="Arm Out") -> ("error out"=w164:errorcluster, "DigitalInputDevRef"=w166:T16)  [unwired: 9 in]
  n160 = call "Lead Screw Control.vi"("Input Velocity"=w105) -> ()  [unwired: 11 in]
  n161 = call <vilib>:"WPI_DigitalInputGetValue.vi"("error in (no error)"=w164, "DigitalInputDevRef"=w166) -> ("Value"=w147:bool)  [unwired: 7 in, 2 out]
  n162 = Less?(x=w130, y=1.5) -> (x < y?=w140:bool)
  n163 = Not(x=w147) -> (.not. x?=w35:bool)
  n164 = Or(x=w140, y=w35) -> (x .or. y?=w139:bool)
  n165 = call <vilib>:"WPI_SolenoidRefNum Registry Get.vi"("refnum name"="Extensions") -> ("SolenoidDevRef"=w142:T21)  [unwired: 9 in, 1 out]
  n166 = call-poly <vilib>:"WPI_SolenoidSet.vi"("Value"=w33, "SolenoidDevRef"=w142) -> ()  [unwired: 8 in, 2 out]
  n167 = call <vilib>:"SD Write Boolean.vi"("Boolean"=w35, "Name"="Arm Out") -> ()  [unwired: 8 in, 2 out]
  n168 = And(x=w143, y=w139) -> (x .and. y?=w154:bool)
  n169 = call <vilib>:"WPI_SolenoidRefNum Registry Get.vi"("refnum name"="Trigger") -> ("error out"=w157:errorcluster, "SolenoidDevRef"=w161:T21)  [unwired: 9 in]
  n170 = call-poly <vilib>:"WPI_SolenoidSet.vi"("error in (no error)"=w157, "Value"=w154, "SolenoidDevRef"=w161) -> ()  [unwired: 7 in, 2 out]
